vi "Init.vi"(8 "error in (no error)":errorcluster, 11 "PongBall in":refnum<class "PongBall.lvclass">) -> (0 "error out":errorcluster, 3 "PongBall out":refnum<class "PongBall.lvclass">)   [LabVIEW 2019, in "RT_Game.lvlib" / "PongBall.lvclass"]
uses:
  PongBall.lvclass
  C:/Users/FreshBob/Dropbox/VIs/myRIO_GameConsole/RT/RT_Game/RT_Sprite/RT_Sprite.lvclass
  C:/Users/FreshBob/Dropbox/VIs/myRIO_GameConsole/RT/RT_Game/GameObject/GameObject.lvclass
  Velocity.ctl
  Engine/Coordinate.ctl
  GameObject/GameObject.lvclass/GameObject.ctl
  PongBall.lvclass/PongBall.ctl
  GameObject/Write MaxSpeed.vi
  GameObject/Write MinSpeed.vi
  GameObject/Write Damping.vi
  GameObject/Write friction.vi
  Write start_pos.vi
  GameObject/Write MaxSpeedX.vi
  GameObject/Write MinSpeedX.vi
  GameObject/Write Velocity.vi
  GameObject/Write IsActive.vi
  GameObject/Write ManualVelocity.vi
  RT_Sprite/RT_Sprite.lvclass
  Engine/Engine.lvclass
  RT_Game.lvlib
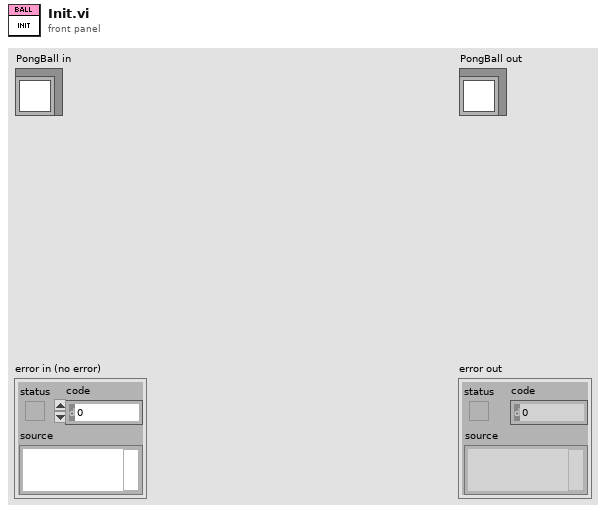
[diagram p1: front panel]
types:
  T1 = typedef "RT_Game.lvlib/Engine.lvclass/Coordinate.ctl" = cluster{"x":dbl, "y":dbl}
  T2 = typedef "RT_Game.lvlib/Velocity.ctl" = cluster{"x":dbl, "y":dbl}
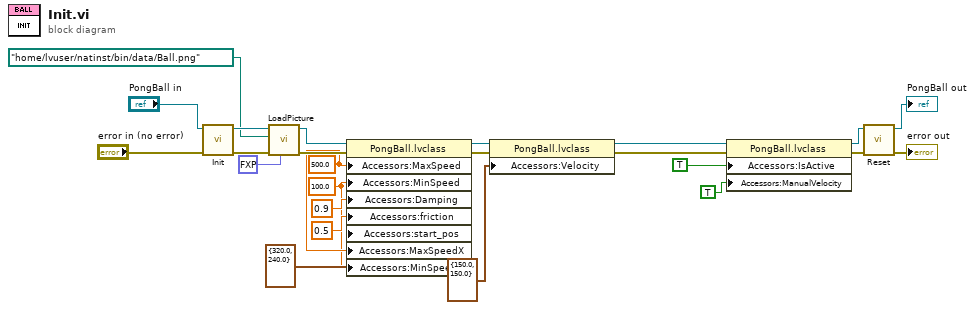
[diagram p0: block diagram]
diagram:
  w1 = 100.0 ("MinSpeed")
  w2 = 500.0 ("MaxSpeed")
  n1 = call-parent "Init.vi"("error in (no error)"="error in (no error)", "RT_Sprite in"="PongBall in") -> ("error out"=w24:errorcluster, "RT_Sprite out"=w20:refnum<class "PongBall.lvclass">)  [unwired: 8 in]
  n2 = call "LoadPicture.vi"("Transparent Color"=fxp<+,3,3> 1.0, "error in (no error)"=w24, "Picture Path"=path "/home/lvuser/natinst/bin/data/Ball.png", "RT_Sprite in"=w20) -> ("error out"=w21:errorcluster, "RT_Sprite out"=w16:refnum<class "PongBall.lvclass">)  [unwired: 6 in]
  n3 = property class="PongBall.lvclass"(reference=w16, error in=w21, "Accessors:MaxSpeed"=w2, "Accessors:MinSpeed"=w1, "Accessors:Damping"=0.9 ("Damping"), "Accessors:friction"=0.5 ("friction"), "Accessors:start_pos"=T1 {"x"=320.0, "y"=240.0} ("start_pos"), "Accessors:MaxSpeedX"=w2, "Accessors:MinSpeedX"=w1) -> (reference out=w6:refnum<class "PongBall.lvclass">, error out=w7:errorcluster)
  n4 = property class="PongBall.lvclass"(reference=w6, error in=w7, "Accessors:Velocity"=T2 {"x"=150.0, "y"=150.0} ("Velocity")) -> (reference out=w13:refnum<class "PongBall.lvclass">, error out=w14:errorcluster)
  n5 = property class="PongBall.lvclass"(reference=w13, error in=w14, "Accessors:IsActive"=TRUE ("IsActive"), "Accessors:ManualVelocity"=TRUE ("ManualVelocity")) -> (reference out=w11:refnum<class "PongBall.lvclass">, error out=w17:errorcluster)
  n6 = call "Reset.vi"("error in (no error)"=w17, "PongBall in"=w11) -> ("error out"=→"error out":errorcluster, "PongBall out"=→"PongBall out":refnum<class "PongBall.lvclass">)  [unwired: 8 in]
